vi "FPGATemperatureResponse.vi"() -> ()   [LabVIEW 2009]
uses:
  <instrlib>/BK Precision 91xx Series/BK Precision 91xx Series.lvlib
panel:
  in  "Array":dbl[](array[numeric])
  out "error out":errorcluster
  in  "VISA resource name":refnum<visa-resource-name>
  in  "Serial Configuration":T1={"Parity(0:none)"=0, "Baud Rate (9600)"=9600, "Data Bits(8)"=8, "Flow Control(None)"=0, " Stop Bits(1.0)"=10} {"Stop Bits(1.0)" items=["1.0"=10, "1.5"=15, "2.0"=20]; "Flow Control(None)" items=["None", "XON/XOFF", "RTS/CTS", "XON/XOFF & RTS/CTS", "DTR/DSR", "XON/XOFF & DTR/DSR"]; "Data Bits(8)" items=["7"=7, "8"=8]; "Baud Rate (9600)" items=["2400"=2400, "4800"=4800, "9600"=9600, "19200"=19200, "38400"=38400]; "Parity(0:none)" items=["None", "Odd", "Even", "Mark", "Space"]}
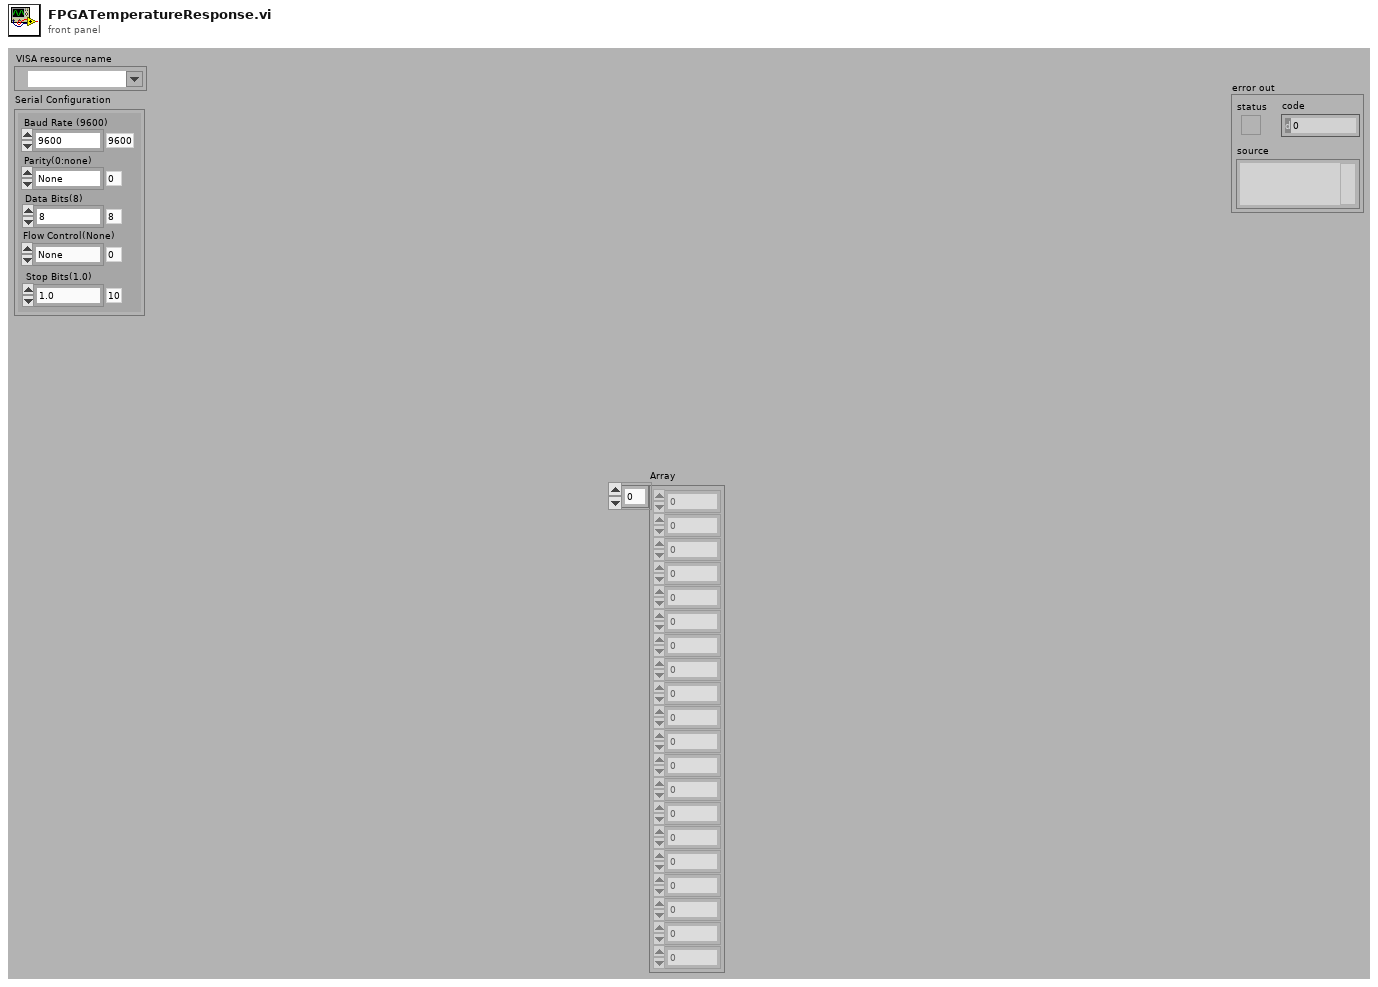
[diagram p1: front panel]
types:
  T1 = cluster{"Parity(0:none)":u16, "Baud Rate (9600)":u16, "Data Bits(8)":u16, "Flow Control(None)":u16, " Stop Bits(1.0)":u16}
  T2 = enum16{"open", "replace", "create", "open or create", "replace or create", "replace or create with confirmation"}
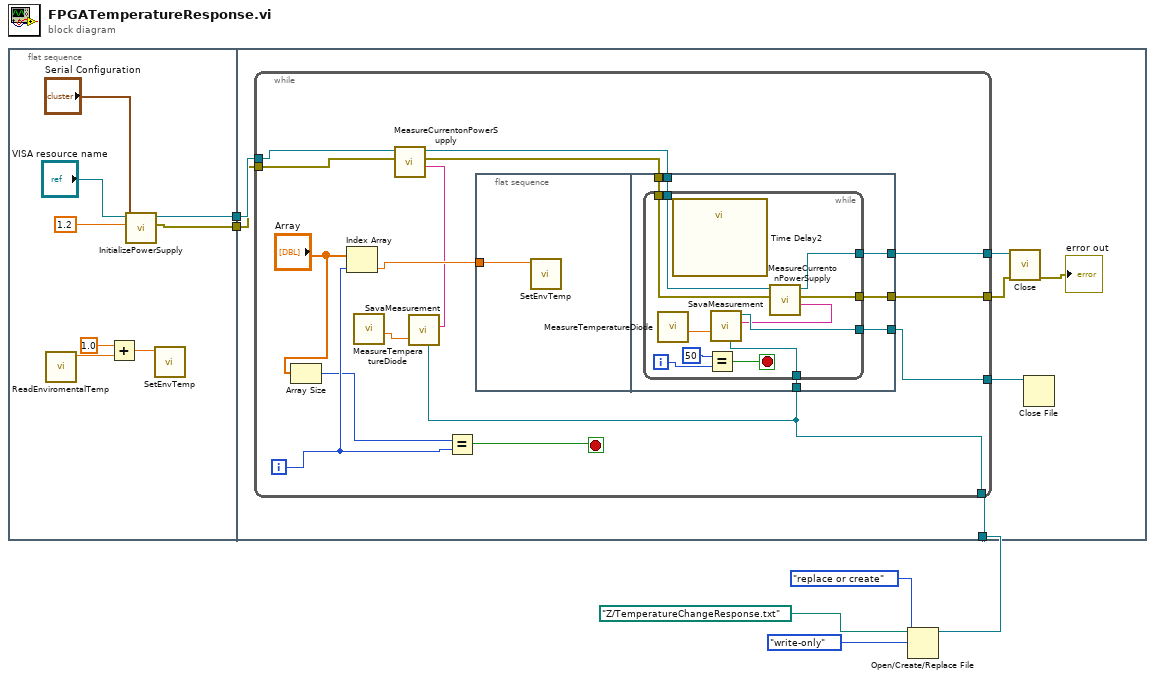
[diagram p0: block diagram]
diagram:
  n1 = flat-sequence {
    tunnel: [w8] -> w6
    tunnel: [w7] -> w5
    tunnel: w1 -> [w20]
    tunnel: w6 -> [w19]
    tunnel: w5 -> [w18]
    frame #0 {
      n2 = call "ReadEnviromentalTemp.vi"() -> ("Probe 1 temperature"=w10:dbl)  [unwired: 10 in, 1 out]
      n3 = Add(x=1.0, y=w10) -> (x+y=w11:dbl)
      n4 = call "InitializePowerSupply.vi"("Serial Configuration"="Serial Configuration", "Manual Range(0.00)"=1.2, "VISA resource name"="VISA resource name") -> ("error out"=w7:errorcluster, "VISA resource name out"=w8:refnum<visa-resource-name>)  [unwired: 7 in]
      n5 = call "SetEnvTemp.vi"("New temperature"=w11) -> ()  [unwired: 10 in, 1 out]
    }
    frame #1 {
      n6 = while {
        tunnel: w20 -> [w22]
        tunnel: w19 -> [w28]
        tunnel: w18 -> [w27]
        tunnel: [w31] -> w17
        tunnel: [w30] -> w16
        tunnel: [w29] -> w15
        i -> [w35]
        stop <- w36 stop-if-true
        n7 = Array Size(array="Array") -> (size(s)=w33:i32)
        n8 = Index Array(array="Array", index=w35) -> (element=w32:dbl)
        n9 = call "MeasureTemperatureDiode.vi"() -> ("Celcius"=w24:dbl)  [unwired: 8 in, 3 out]
        n10 = call "MeasureCurrentonPowerSupply.vi"("error in (no error)"=w27, "VISA resource name"=w28) -> ("Measurement"=w23:string, "error out"=w25:errorcluster, "VISA resource name out"=w26:refnum<visa-resource-name>)  [unwired: 7 in]
        n11 = call "SavaMeasurement.vi"("Measurement"=w23, "refnum out"=w22, "DiodeTemperature"=w24) -> ()  [unwired: 2 in, 2 out]
        n12 = Equal?(x=w33, y=w35) -> (x = y?=w36:bool)
        n13 = flat-sequence {
          tunnel: w32 -> [w37]
          tunnel: [w43] -> w29
          tunnel: w26 -> [w42]
          tunnel: w25 -> [w41]
          tunnel: [w40] -> w31
          tunnel: [w39] -> w30
          tunnel: w22 -> [w38]
          frame #0 {
            n14 = call "SetEnvTemp.vi"("New temperature"=w37) -> ()  [unwired: 10 in, 1 out]
          }
          frame #1 {
            n15 = while {
              tunnel: [w50] -> w43
              tunnel: w42 -> [w48]
              tunnel: w41 -> [w47]
              tunnel: [w46] -> w40
              tunnel: [w45] -> w39
              tunnel: w38 -> [w44]
              i -> [w53]
              stop <- w51 stop-if-true
              n16 = call "MeasureTemperatureDiode.vi"() -> ("Celcius"=w54:dbl)  [unwired: 8 in, 3 out]
              n17 = call "Time Delay2"() -> ()  [unwired: 11 in, 1 out]
              n18 = Equal?(x=50, y=w53) -> (x = y?=w51:bool)
              n19 = call "MeasureCurrentonPowerSupply.vi"("error in (no error)"=w47, "VISA resource name"=w48) -> ("Measurement"=w49:string, "error out"=w45:errorcluster, "VISA resource name out"=w46:refnum<visa-resource-name>)  [unwired: 7 in]
              n20 = call "SavaMeasurement.vi"("Measurement"=w49, "refnum out"=w44, "DiodeTemperature"=w54) -> ("refnum out 2"=w50:refnum<file>)  [unwired: 2 in, 1 out]
            }
          }
        }
      }
      n21 = call <instrlib>:"Close.vi"("error in (no error)"=w16, "VISA resource name"=w17) -> ("error out"=→"error out":errorcluster)  [unwired: 9 in]
      n22 = Close File(refnum=w15) -> ()  [unwired: 1 in, 2 out]
    }
  }
  n23 = Open/Create/Replace File(file path (use dialog)=path "Z:/TemperatureChangeResponse.txt", operation (0:open)=T2."replace or create", access (0:read/write)=enum16{"read/write", "read-only", "write-only"}."write-only") -> (refnum out=w1:refnum<file>)  [unwired: 3 in, 2 out]
